vi "globalTearDown.vi"(8 "error in (no error)":errorcluster, 11 "testcase-CSMGlobalLog in":refnum<class "testcase-CSMGlobalLog.lvclass">) -> (0 "error out":errorcluster, 3 "testcase-CSMGlobalLog out":refnum<class "testcase-CSMGlobalLog.lvclass">)   [LabVIEW 2017, in "testcase-CSMGlobalLog.lvclass"]
uses:
  testcase-CSMGlobalLog.lvclass
  GlobalVariable.vi
  src/user.lib/_NEVSTOP/Communicable State Machine(CSM)/Communicable State Machine.lvlib
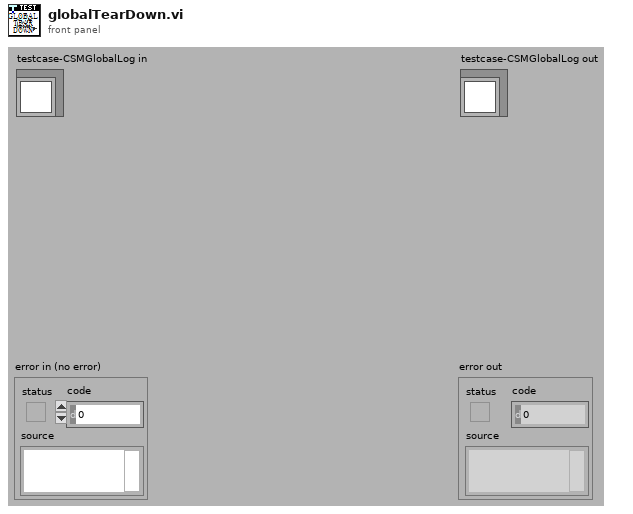
[diagram p1: front panel]
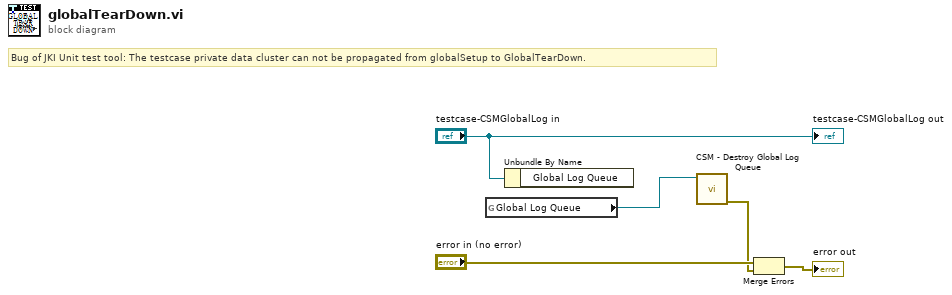
[diagram p0: block diagram]
diagram:
  # "Bug of JKI Unit test tool: The testcase private data cluster can not be propagated from globalSetup to GlobalTearDown."
  n1 = global read "GlobalVariable.vi" "Global Log Queue"() -> (w1:refnum<queue>)
  n2 = Unbundle By Name("testcase-CSMGlobalLog in") -> ()  [unwired: 1 out]
  n3 = call "CSM - Destroy Global Log Queue.vi"("Global Log Queue"=w1) -> ("error out"=w2:errorcluster)  [unwired: 10 in]
  n4 = Merge Errors("error in (no error)", w2) -> (→"error out":errorcluster)
  "testcase-CSMGlobalLog out" <- "testcase-CSMGlobalLog in"
